vi "endAD.vi"(0 "设备":dbl) -> ()   [LabVIEW 2018]
uses:
  main/PCI8552B_32.dll
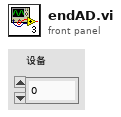
[diagram p1: front panel]
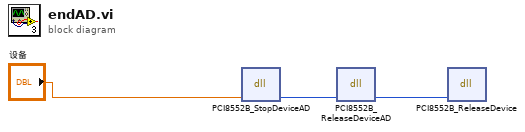
[diagram p0: block diagram]
diagram:
  n1 = dll-call lib="PTH2…abs E\nPersonal Fileç ”ç©¶ç”Ÿå­¦ä¹ 202002-202007ç ”ä¸€ä¸‹å­¦æœŸwork2020\nSARControllerSAR-ControllermainPCI8552B_32.DLL" fn="PCI8552B_StopDeviceAD" label="StopDeviceAD"("hDevice"="设备") -> ("hDevice"=w3:i32)  [unwired: 4 in, 2 out]
  n2 = dll-call lib="PTH2…abs E\nPersonal Fileç ”ç©¶ç”Ÿå­¦ä¹ 202002-202007ç ”ä¸€ä¸‹å­¦æœŸwork2020\nSARControllerSAR-ControllermainPCI8552B_32.DLL" fn="PCI8552B_ReleaseDeviceAD" label="ReleaseDeviceAD"("hDevice"=w3) -> ("hDevice"=w2:i32)  [unwired: 4 in, 2 out]
  n3 = dll-call lib="PTH2…abs E\nPersonal Fileç ”ç©¶ç”Ÿå­¦ä¹ 202002-202007ç ”ä¸€ä¸‹å­¦æœŸwork2020\nSARControllerSAR-ControllermainPCI8552B_32.DLL" fn="PCI8552B_ReleaseDevice" label="ReleaseDevice"("hDevice"=w2) -> ()  [unwired: 5 in, 2 out]
